vi "XY Plot - Title--Const.vi"() -> (3 "XY Plot Title":string)   [LabVIEW 2017, in "DTacq Plot Display Library.lvlib"]
uses:
  DTacq Plot Display Library.lvlib
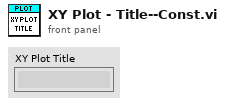
[diagram p1: front panel]
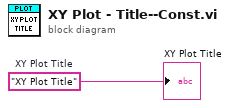
[diagram p0: block diagram]
diagram:
  w1 = "XY Plot Title"  # XY Plot Title
  "XY Plot Title" <- w1
